vi "Get Temperature - Multiple.vi"(0 "reference in":refnum<class "Temp.lvclass">, 3 "Temperature Channel Numbers (Zero Based)":i32[](array[numeric])=[0, 1, 2, 3], 5 "error in (no error)":errorcluster) -> (14 "reference out":refnum<class "Temp.lvclass">, 16 "Temperature Channel Readings":dbl[](array[numeric]), 17 "Temperature Average Among Channels":dbl, 18 "Temperature Standard Deviation Among Channels":dbl, 19 "error out":errorcluster)   [LabVIEW 2017, in "Temp.lvclass"]
uses:
  Temp.lvclass
  <vilib>/Analysis/NI_AALBase.lvlib
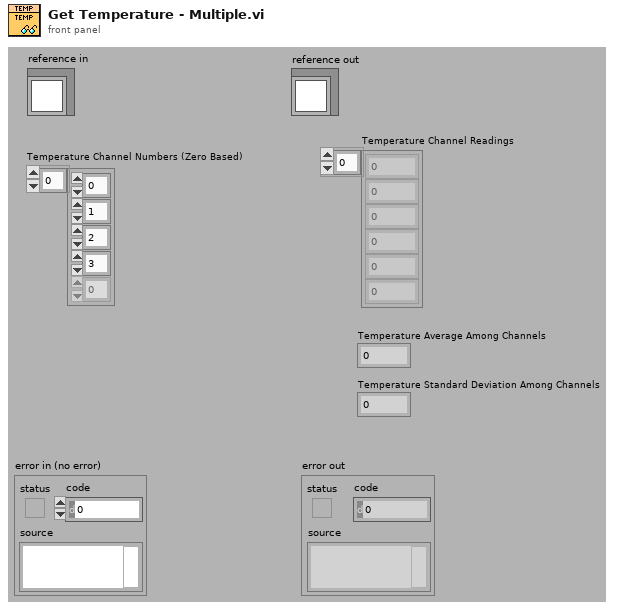
[diagram p1: front panel]
types:
  T1 = typedef "Temp.lvclass/ObjectAttributes.ctl" = cluster{"Temperature Task":refnum<k21>, "Temperature Readings":dbl[], "Thermocouple Type":i32, "Temperature Units":i32, "Average Temperature":dbl, "Number of Temperature Modules":i32, "Number of Total Temperature Channels":i32, "Temperature On/Off Status":bool, "Temperature Module Names (NI-Max Name)":string[], "Number of Channels Per Temperature  Module":i32[], "Temperature VI Reference":refnum<vi>}
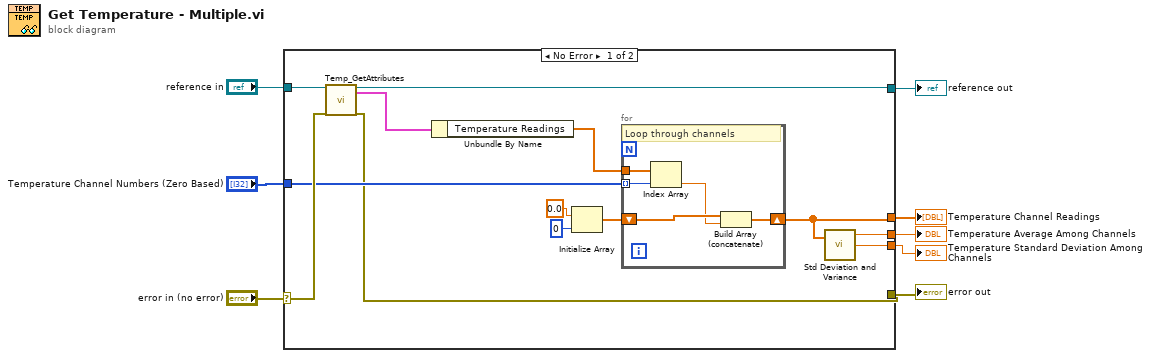
[diagram p0: block diagram]
diagram:
  n1 = case shown="No Error" "error in (no error)" {
    selector: "error in (no error)" -> [w20 w28]
    tunnel: [w14 w28] -> w7
    tunnel: [w19 w27] -> w5
    tunnel: "reference in" -> [w21 w27]
    tunnel: "Temperature Channel Numbers (Zero Based)" -> [w18 _]
    tunnel: [w17 _] -> w3
    tunnel: [w16 _] -> w2
    tunnel: [w15 _] -> w1
    frame No Error {
      n2 = call "Temp_GetAttributes.vi"("reference in"=w21, "error in (no error)"=w20) -> ("reference out"=w19:refnum<class "Temp.lvclass">, "Data"=w9:T1, "error out"=w14:errorcluster)  [unwired: 14 in, 1 out]
      n3 = Unbundle By Name(w9) -> ("Temperature Readings"=w13:dbl[])
      n4 = Initialize Array(0.0 ("element"), 0 ("dimension size")) -> (w10:dbl[])
      n5 = for {
        tunnel: w18 -> [w25] mode=indexing
        tunnel: w13 -> [w26]
        shift-right: [w23] -> w17
        shift-left: w10 -> [w24]
        # "Loop through channels"
        n6 = Index Array(array=w26, index=w25) -> (element=w22:dbl)
        n7 = Build Array (concatenate)(w24, w22) -> (w23:dbl[])
      }
      n8 = call <vilib>:"Std Deviation and Variance.vi"("X"=w17) -> ("mean"=w15:dbl, "standard deviation"=w16:dbl)  [unwired: 1 in, 1 out]
    }
    frame Error {
    }
  }
  "error out" <- w7
  "reference out" <- w5
  "Temperature Channel Readings" <- w3
  "Temperature Average Among Channels" <- w1
  "Temperature Standard Deviation Among Channels" <- w2
